vi "get sequence action by index.vi"(8 "error in (no error)":errorcluster, 9 "index":i32, 10 "sequence name":string, 11 "Simple Sequencer TBM configuration in":refnum<class "Simple Sequencer TBM configuration.lvclass">) -> (0 "error out":errorcluster, 2 "action configuration":refnum<class "action configuration.lvclass">, 3 "Simple Sequencer TBM configuration out":refnum<class "Simple Sequencer TBM configuration.lvclass">)   [LabVIEW 2014, in "Simple Sequencer TBM configuration.lvclass"]
doc: "If you pass in a Sequence Name and an Index in that sequence, this VI will return the corresponding Action configuration object at that location."
uses:
  Simple Sequencer TBM configuration.lvclass
  sequencer parent classes/action configuration parent/action configuration.lvclass
  Simple Sequencer TBM configuration.lvclass/Simple Sequencer TBM configuration.ctl
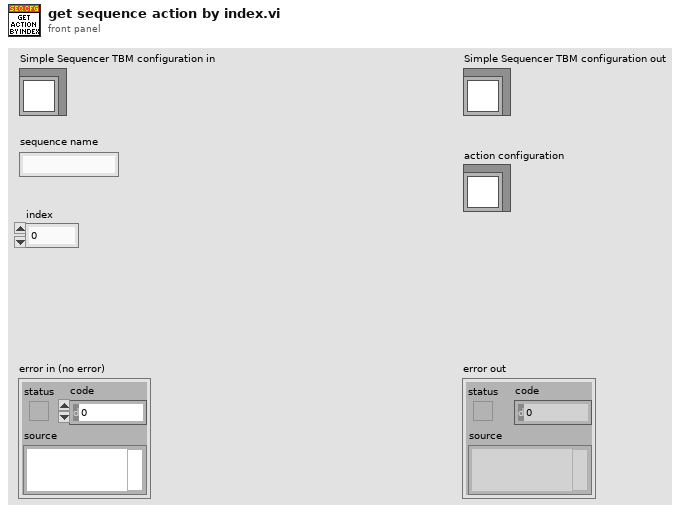
[diagram p1: front panel]
types:
  T1 = typedef "Simple Sequencer TBM configuration.lvclass/sequence definition.ctl" = cluster{"sequence name":string, "action configs":refnum<class "action configuration.lvclass">[]}
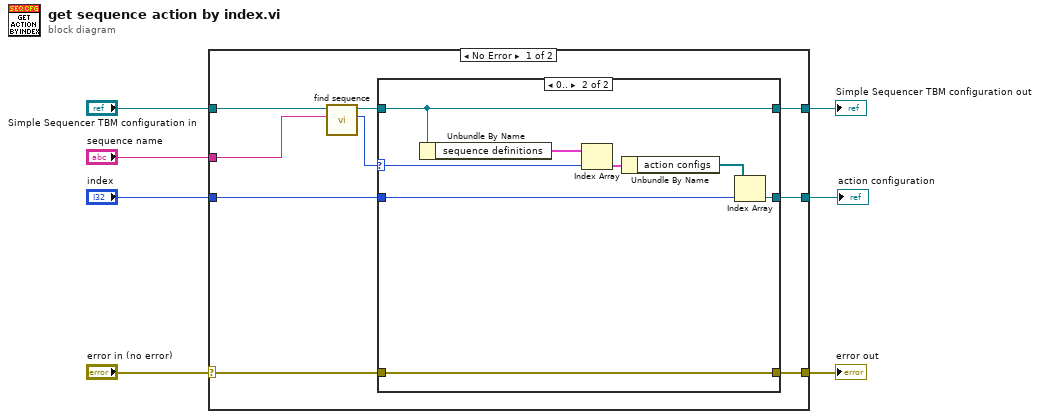
[diagram p0: block diagram]
diagram:
  n1 = case shown="No Error" "error in (no error)" {
    selector: "error in (no error)" -> [w12 w28]
    tunnel: [w11 w28] -> w6
    tunnel: [w10 w27] -> w4
    tunnel: "Simple Sequencer TBM configuration in" -> [w16 w27]
    tunnel: "sequence name" -> [w15 _]
    tunnel: "index" -> [w9 _]
    tunnel: [w8 _] -> w1
    frame No Error {
      n2 = call "find sequence.vi"("sequence name"=w15, "Simple Sequencer TBM configuration in"=w16) -> ("index"=w13:i32, "Simple Sequencer TBM configuration out"=w14:refnum<class "Simple Sequencer TBM configuration.lvclass">)  [unwired: 8 in]
      n3 = case shown="0.." w13 {
        selector: w13 -> [_ w24]
        tunnel: w14 -> [w17 w23]
        tunnel: w12 -> [w18 w25]
        tunnel: [w18 w25] -> w11
        tunnel: [w17 w23] -> w10
        tunnel: w9 -> [_ w20]
        tunnel: [_ w19] -> w8
        frame ..-1 {
          # "#todo throw error not found"
        }
        frame 0.. {
          n4 = Unbundle By Name(w23) -> ("sequence definitions"=w26:T1[])
          n5 = Index Array(array=w26, index=w24) -> (element=w22:T1)
          n6 = Unbundle By Name(w22) -> ("action configs"=w21:refnum<class "action configuration.lvclass">[])
          n7 = Index Array(array=w21, index=w20) -> (element=w19:refnum<class "action configuration.lvclass">)
        }
      }
    }
    frame Error {
    }
  }
  "error out" <- w6
  "Simple Sequencer TBM configuration out" <- w4
  "action configuration" <- w1
